vi "Compute one line from two straight edge lines.vi"(11 "Straight Edges":T1(array[cluster]) {"Point2 (Real-World)"."Y" format="%.2f"; "Point2 (Real-World)"."X" format="%.2f"; "Point1 (Real-World)"."Y" format="%.2f"; "Point1 (Real-World)"."X" format="%.2f"; "Point2 (Pixels)"."Y" format="%.2f"; "Point2 (Pixels)"."X" format="%.2f"; "Point1 (Pixels)"."Y" format="%.2f"; "Point1 (Pixels)"."X" format="%.2f"}) -> (0 "Y":sgl, 1 "delta y = 0, slope 0":bool, 2 "intercept":dbl, 3 "slope":dbl)   [LabVIEW 2017]
uses:
  <vilib>/Analysis/baseanly.llb/Mean (DBL).vi
  <vilib>/Analysis/NI_AALBase.lvlib
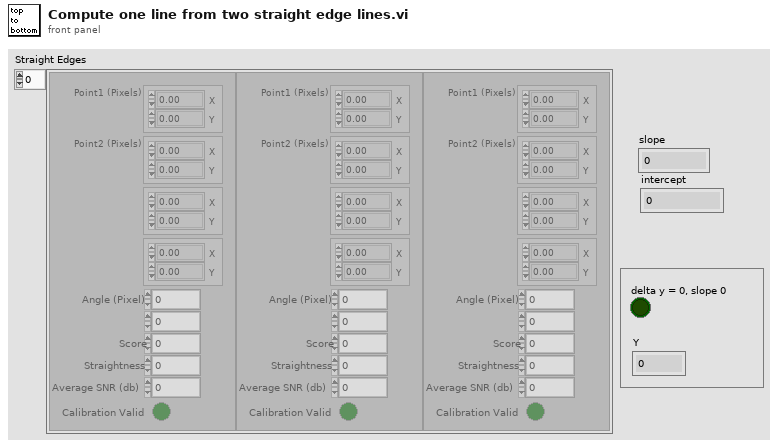
[diagram p1: front panel]
types:
  T1 = cluster{"Point1 (Pixels)":cluster{"X":sgl, "Y":sgl}, "Point2 (Pixels)":cluster{"X":sgl, "Y":sgl}, "Point1 (Real-World)":cluster{"X":sgl, "Y":sgl}, "Point2 (Real-World)":cluster{"X":sgl, "Y":sgl}, "Angle (Pixel)":dbl, "Angle (Real-World)":dbl, "Score":dbl, "Straightness":dbl, "Average SNR (db)":dbl, "Calibration Valid":bool}[]
  T2 = cluster{"Point1 (Pixels)":cluster{"X":sgl, "Y":sgl}, "Point2 (Pixels)":cluster{"X":sgl, "Y":sgl}, "Point1 (Real-World)":cluster{"X":sgl, "Y":sgl}, "Point2 (Real-World)":cluster{"X":sgl, "Y":sgl}, "Angle (Pixel)":dbl, "Angle (Real-World)":dbl, "Score":dbl, "Straightness":dbl, "Average SNR (db)":dbl, "Calibration Valid":bool}
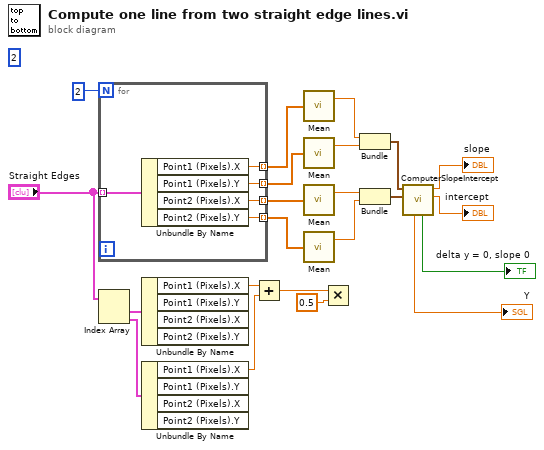
[diagram p0: block diagram]
diagram:
  (unwired) 2
  n1 = for {
    N: 2 -> [_]
    tunnel: "Straight Edges" -> [w27] mode=indexing
    tunnel: [w26] -> w13 mode=indexing
    tunnel: [w25] -> w12 mode=indexing
    tunnel: [w24] -> w11 mode=indexing
    tunnel: [w23] -> w10 mode=indexing
    n2 = Unbundle By Name(w27) -> ("Point1 (Pixels).X"=w26:sgl, "Point1 (Pixels).Y"=w25:sgl, "Point2 (Pixels).X"=w24:sgl, "Point2 (Pixels).Y"=w23:sgl)
  }
  n3 = Index Array(array="Straight Edges") -> (element #1=w18:T2, element #2=w17:T2)  [unwired: 2 in]
  n4 = Unbundle By Name(w18) -> ("Point1 (Pixels).X"=w21:sgl)  [unwired: 3 out]
  n5 = Unbundle By Name(w17) -> ("Point1 (Pixels).X"=w16:sgl)  [unwired: 3 out]
  n6 = Add(x=w21, y=w16) -> (x+y=w20:sgl)
  n7 = call-poly <vilib>:"Mean.vi"("X"=w13) -> ("mean"=w9:dbl)  [unwired: 1 out]
  n8 = call-poly <vilib>:"Mean.vi"("X"=w12) -> ("mean"=w8:dbl)  [unwired: 1 out]
  n9 = call-poly <vilib>:"Mean.vi"("X"=w11) -> ("mean"=w6:dbl)  [unwired: 1 out]
  n10 = call-poly <vilib>:"Mean.vi"("X"=w10) -> ("mean"=w5:dbl)  [unwired: 1 out]
  n11 = Multiply(x=w20, y=sgl 0.5) -> ()  [unwired: 1 out]
  n12 = Bundle("mean"=w9, "mean"=w8) -> (w7:cluster{"mean":dbl, "mean":dbl})  [unwired: 1 in]
  n13 = Bundle("mean"=w6, "mean"=w5) -> (w4:cluster{"mean":dbl, "mean":dbl})  [unwired: 1 in]
  n14 = call "ComputerSlopeIntercept.vi"("Point2 (Pixels)"=w4, "Point1 (Pixels)"=w7) -> ("intercept"=→"intercept":dbl, "slope"=→"slope":dbl, "delta y = 0, slope 0"=→"delta y = 0, slope 0":bool, "Y"=→"Y":sgl)  [unwired: 4 in, 2 out]
